vi "Test1.vi"() -> ()   [LabVIEW 2010]
uses:
  <vilib>/MDSplus/Classes/Data_Class/Scalar_Class/Float32_Class/Float32.lvclass
panel:
  out "Float out":sgl
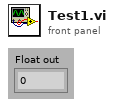
[diagram p1: front panel]
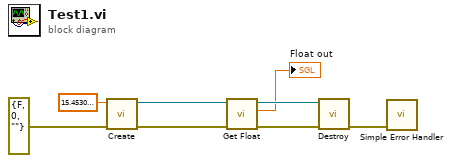
[diagram p0: block diagram]
diagram:
  n1 = call <vilib>:"Create.vi"("error in (no error)"=errorcluster {"status"=FALSE, "code"=0, "source"=""}, "SGL in"=sgl 15.453 ("Value")) -> ("error out"=w6:errorcluster, "Float32 out"=w8:refnum<class "Float32.lvclass">)  [unwired: 8 in]
  n2 = call-dynamic "Get Float.vi"("error in (no error)"=w6, "Float32 in"=w8) -> ("error out"=w4:errorcluster, "SGL out"=→"Float out":sgl, "Float32 out"=w5:refnum<class "Float32.lvclass">)  [unwired: 7 in]
  n3 = call-dynamic "Destroy.vi"("error in (no error)"=w4, "Float32 in"=w5) -> ("error out"=w3:errorcluster)  [unwired: 9 in]
  n4 = call <vilib>:"Simple Error Handler.vi"("error in (no error)"=w3) -> ()  [unwired: 4 in, 5 out]
